vi "_Measure 1 Period TF.vi"() -> ()   [LabVIEW 2014]
panel:
  out "elemszam korlat":dbl
  out "real fs [Hz]":dbl
  out "Waveform Graph":waveform(dbl)[](graph)
  out "Phase":dbl
  out "Mag":dbl
  out "tmr 2 rld value":u16
  in  "Signal freq [Hz]":dbl=1000.0
  in  "Elemszam":u8
  out "VISA Refnum out":refnum<visa-resource-name>
  out "error out":errorcluster
  in  "VISA Refnum in":refnum<visa-resource-name>
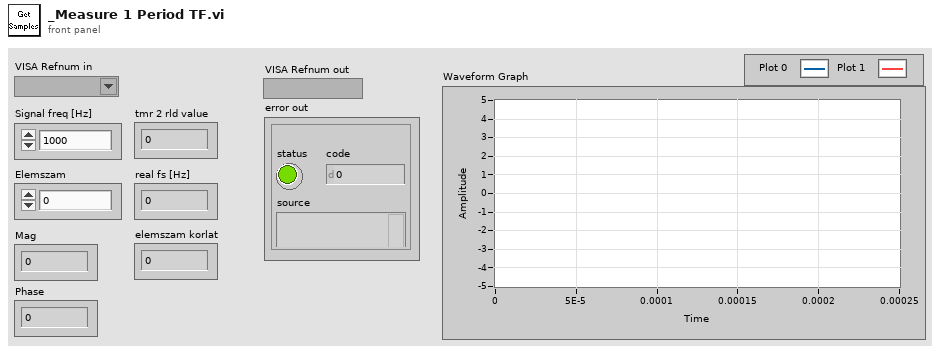
[diagram p1: front panel]
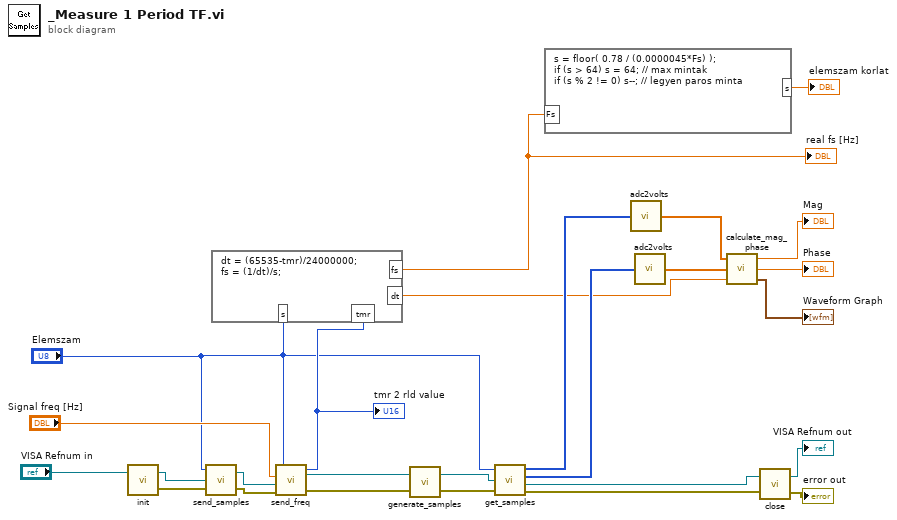
[diagram p0: block diagram]
diagram:
  n1 = call "init.vi"("VISA Refnum in"="VISA Refnum in") -> ("error out"=w15:errorcluster, "VISA Refnum out"=w16:refnum<visa-resource-name>)  [unwired: 1 in]
  n2 = call "send_samples.vi"("error in (no error)"=w15, "VISA Refnum in"=w16, "elemszam"="Elemszam") -> ("error out"=w13:errorcluster, "VISA Refnum out"=w14:refnum<visa-resource-name>)
  n3 = call "send_freq.vi"("error in (no error)"=w13, "VISA Refnum in"=w14, "signal freq"="Signal freq [Hz]", "elemszam"="Elemszam") -> ("error out"=w22:errorcluster, "VISA Refnum out"=w21:refnum<visa-resource-name>, "tmr 2 rld value"=w3:u16)
  "tmr 2 rld value" <- w3
  n4 = formula code="dt = (65535-tmr)/24000000;\nfs = (1/dt)/s;"("tmr"=w3, "s"="Elemszam") -> ("dt"=w1:dbl, "fs"=w4:dbl)
  "real fs [Hz]" <- w4
  n5 = call "generate_samples.vi"("error in (no error)"=w22, "VISA Refnum in"=w21) -> ("error out"=w23:errorcluster, "VISA Refnum out"=w17:refnum<visa-resource-name>)
  n6 = call "get_samples.vi"("elemszam"="Elemszam", "VISA Refnum in"=w17, "error in (no error)"=w23) -> ("in samples"=w12:u16[], "out samples"=w11:u16[], "VISA Refnum out"=w18:refnum<visa-resource-name>, "error out"=w20:errorcluster)
  n7 = formula code="s = floor( 0.78 / (0.0000045*Fs) );\nif (s > 64) s = 64; // max mintak\nif (s % 2 != 0) s--; // legyen paros minta"("Fs"=w4) -> ("s"=→"elemszam korlat":dbl)
  n8 = call "adc2volts.vi"("ADC value"=w12) -> ("Volts"=w9:dbl[])
  n9 = call "adc2volts.vi"("ADC value"=w11) -> ("Volts"=w8:dbl[])
  n10 = call "calculate_mag_phase.vi"("dt"=w1, "OUT samples"=w8, "IN samples"=w9) -> ("Measured Signals"=→"Waveform Graph":waveform(dbl)[], "Phase"=→"Phase":dbl, "Magnitude"=→"Mag":dbl)
  n11 = call "close.vi"("error in (no error)"=w20, "VISA resource name"=w18) -> ("error out"=→"error out":errorcluster, "VISA resource name out"=→"VISA Refnum out":refnum<visa-resource-name>)
